vi "Title-Change.vi"(1 "Parameters":variant, 2 "New Title":string, 3 "Index":i32) -> (0 "Variant":variant)   [LabVIEW 2019]
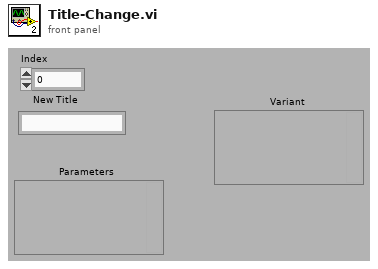
[diagram p1: front panel]
types:
  T1 = typedef "Instrument Properties.ctl" = cluster{"Public":T2, "Private":T3}
  T2 = typedef "Public.ctl" = cluster{"Column Name":string[], "Trace Color":u32[]}
  T3 = typedef "Private.ctl" = cluster{"Path":path, "VI Refnum":T4, "Name":string, "# of Values":i32, "Scale Factors":dbl[], "Display":T5[], "Offset":dbl[]}
  T4 = typedef "Instrument Ref.ctl" = refnum<vi>
  T5 = typedef "SystemCheckBox-resize.ctl" = bool
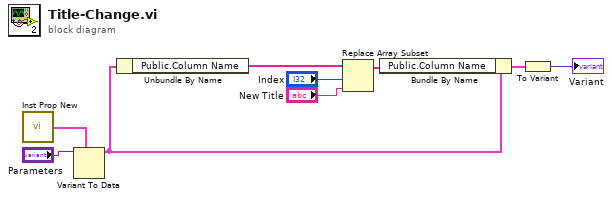
[diagram p0: block diagram]
diagram:
  n1 = call "Inst Prop New.vi"() -> ("Instrument Prop Out"=w7:T1)
  n2 = Variant To Data(type=w7, Variant="Parameters") -> (data=w5:T1)  [unwired: 1 in, 1 out]
  n3 = Unbundle By Name(w5) -> ("Public.Column Name"=w4:string[])
  n4 = Replace Array Subset(array=w4, new element="New Title", index="Index") -> (w6:string[])
  n5 = Bundle By Name(cluster=w5, "Public.Column Name"=w6) -> (w3:T1)
  n6 = To Variant(anything=w3) -> (Variant=→"Variant":variant)
